vi "Add Test Parameter.vi"(7 "Data Value ID":string, 8 "error in (no error)":errorcluster, 10 "Data Value":variant, 11 "Test in":refnum<class "Test.lvclass">) -> (0 "error out":errorcluster, 3 "Test out":refnum<class "Test.lvclass">)   [LabVIEW 2018, in "Test.lvclass"]
uses:
  Test.lvclass
  Test.lvclass/Test.ctl
  78035fa3-d753-4dfc-b146-cd1640418e3a.vi
  d0fcabb1-b984-4c0c-aac6-ca8934018952.vi
  <vilib>/JDP Science/JSONtext/Variant to JSON Text.vi
  <vilib>/JDP Science/JSONtext/JSONtext.lvlib
  <vilib>/Utility/Data Type/NI_Data Type.lvlib
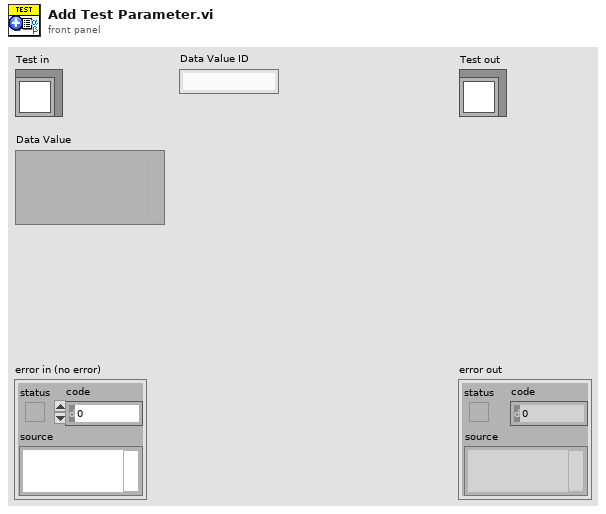
[diagram p1: front panel]
types:
  T1 = typedef "NI_Data Type.lvlib/Data Type.ctl" = enum8{"Invalid Type", "Void", "I8", "I16", "I32", "I64", "U8", "U16", "U32", "U64", "Single Float", "Double Float", "Extended Float", "Single Complex", "Double Complex", "Extended Complex", "Enum U8", "Enum U16", "Enum U32", "Enum U64", "Single Float With Unit", "Double Float With Unit", "Extended Float With Unit", "Single Complex with Unit", "Double Complex with Unit", "Extended Complex with Unit", "Boolean", "String", "Path", "Picture", "Tag", "Array", "Cluster", "Variant", "LV Variant", "Waveform", "Timestamp", "Digital Waveform", "Digital Data", "ExpressData", "Refnum", "External Data", "VI", "Poly VI", "LabVIEW Class Instance", "Fixed Point"}
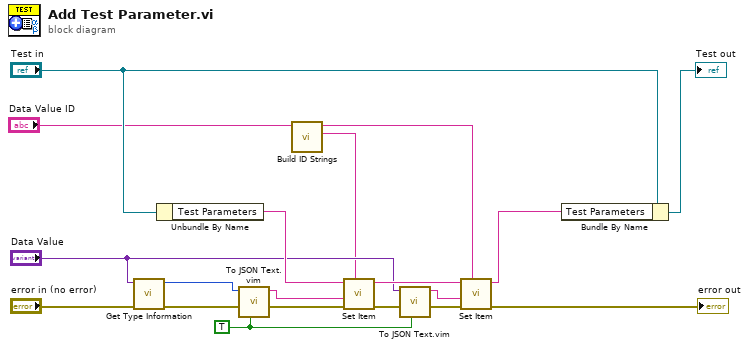
[diagram p0: block diagram]
diagram:
  w1 = TRUE ("Pretty Print?")
  n1 = call <vilib>:"Get Type Information.vi"("error in (no error)"="error in (no error)", "Variant"="Data Value") -> ("error out"=w14:errorcluster, "Type"=w12:T1)  [unwired: 5 in, 3 out]
  n2 = Unbundle By Name("Test in") -> ("Test Parameters"=w16:string)
  n3 = call "To JSON Text.vim"("Pretty Print?"=w1, "error in (no error)"=w14, "Anything"=w12) -> ("error out"=w13:errorcluster, "<JSON>"=w11:string)  [unwired: 7 in]
  n4 = call "Build ID Strings.vi"("Data Value ID"="Data Value ID") -> ("Type ID"=w3:string, "Value ID"=w2:string)  [unwired: 9 in]
  n5 = call <vilib>:"Set Item.vi"("$Path or Item Name"=w3, "error in (no error)"=w13, "JSON to Insert"=w11, "JSON"=w16) -> ("error out"=w18:errorcluster, "<JSON>"=w8:string)  [unwired: 4 in, 1 out]
  n6 = call "To JSON Text.vim"("Pretty Print?"=w1, "error in (no error)"=w18, "Anything"="Data Value") -> ("error out"=w10:errorcluster, "<JSON>"=w5:string)  [unwired: 7 in]
  n7 = call <vilib>:"Set Item.vi"("$Path or Item Name"=w2, "error in (no error)"=w10, "JSON to Insert"=w5, "JSON"=w8) -> ("error out"=→"error out":errorcluster, "<JSON>"=w7:string)  [unwired: 4 in, 1 out]
  n8 = Bundle By Name(cluster="Test in", "Test Parameters"=w7) -> (→"Test out":refnum<class "Test.lvclass">)
